vi "IsStayModeOP.vi"(8 "errin":errorcluster) -> (0 "errout":errorcluster, 3 "OK?":bool)   [LabVIEW 2020]
doc: "Mode DRIVE sur 10s OK? sans DTC?"
uses:
  10-ZEN35-PkOp/SubVi/VG 106 STATUS.vi
panel:
  out "F106 Power Distribution Status":string
  out "F106 Operating Status":string
  out "F106 Battery State":string
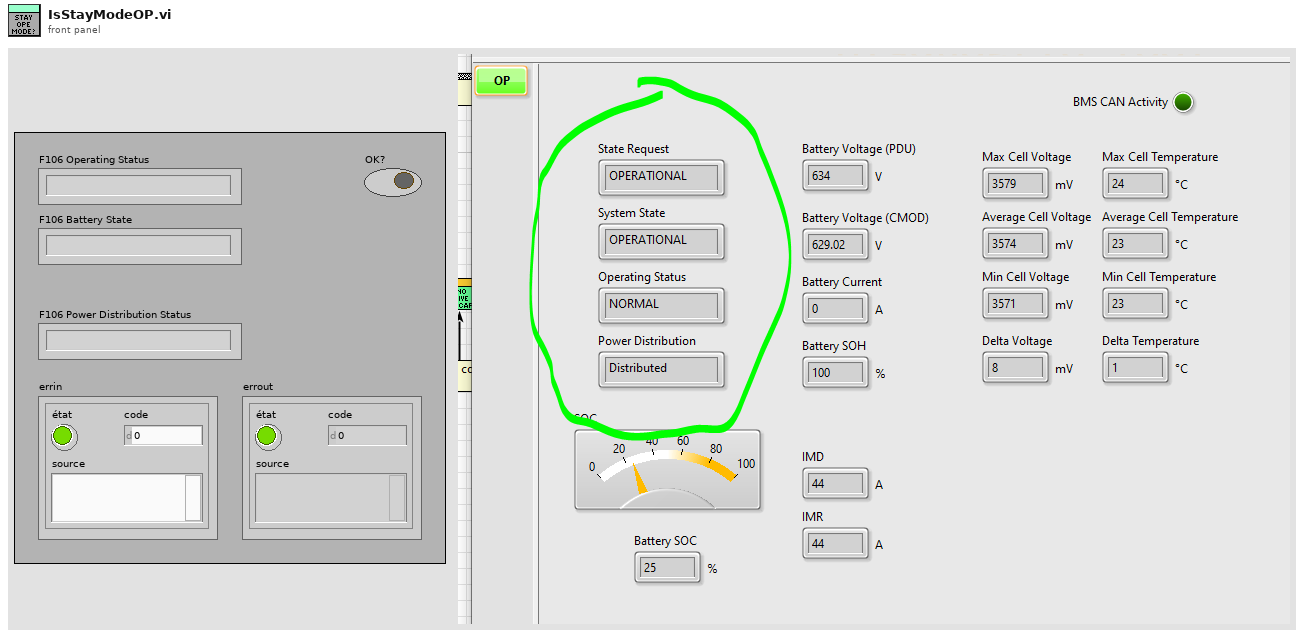
[diagram p1: front panel]
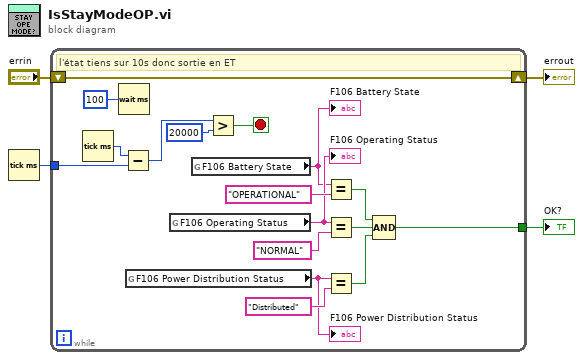
[diagram p0: block diagram]
diagram:
  n1 = Tick Count (ms)() -> (millisecond timer value=w1:u32)
  n2 = while {
    shift-right: [w21] -> w4
    shift-left: "errin" -> [w21]
    tunnel: w1 -> [w13]
    tunnel: [w10] -> w2
    stop <- w5 stop-if-true
    # "l'état tiens sur 10s donc sortie en ET"
    n3 = Tick Count (ms)() -> (millisecond timer value=w14:u32)
    n4 = Wait (ms)(milliseconds to wait=u32 100 ("attente (ms)")) -> ()  [unwired: 1 out]
    n5 = Subtract(x=w14, y=w13) -> (x-y=w12:u32)
    n6 = global read "VG 106 STATUS.vi" "F106 Power Distribution Status"() -> (w6:string)
    "F106 Power Distribution Status" <- w6
    n7 = global read "VG 106 STATUS.vi" "F106 Operating Status"() -> (w8:string)
    "F106 Operating Status" <- w8
    n8 = global read "VG 106 STATUS.vi" "F106 Battery State"() -> (w7:string)
    "F106 Battery State" <- w7
    n9 = Greater?(x=w12, y=u32 20000) -> (0:w5:bool)
    n10 = Equal?(x=w7, y="OPERATIONAL") -> (x = y?=w17:bool)
    n11 = Equal?(x=w8, y="NORMAL") -> (x = y?=w16:bool)
    n12 = Equal?(x=w6, y="Distributed") -> (x = y?=w15:bool)
    n13 = Compound Arithmetic op=AND(w17, w16, w15) -> (w10:bool)
  }
  "errout" <- w4
  "OK?" <- w2
